vi "APcorrect.vi"(5 "EN_AP":dbl, 7 "c":dbl[](array[numeric]), 8 "error in":errorcluster, 10 "inputData":cdb[](array[numeric]), 11 "Path In":path) -> (0 "error out":errorcluster, 2 "out_data":cdb[](array[numeric]), 3 "Path Out":path)   [LabVIEW 2015]
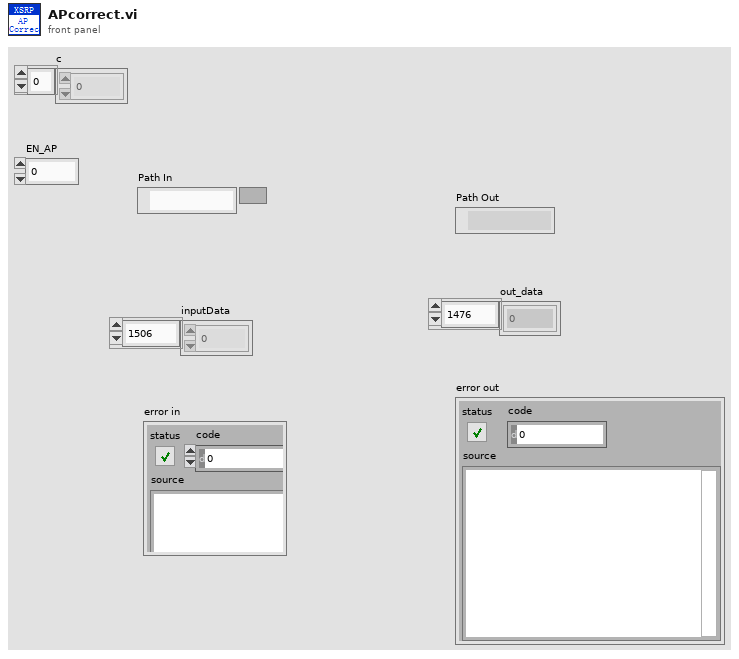
[diagram p1: front panel]
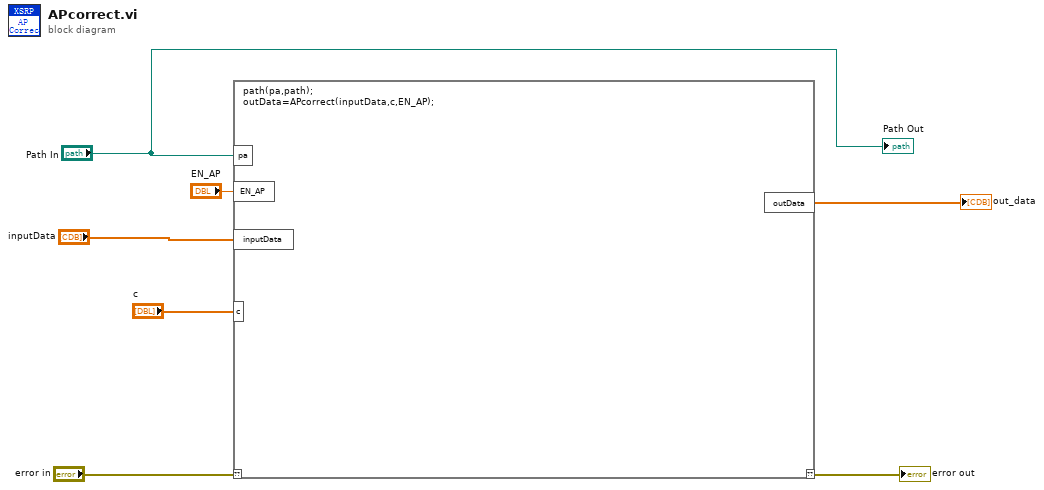
[diagram p0: block diagram]
diagram:
  n1 = script code="path(pa,path);\noutData=APcorrect(inputData,c,EN_AP);"("??"="error in", "pa"="Path In", "inputData"="inputData", "c"="c", "EN_AP"="EN_AP") -> ("??"=→"error out":errorcluster, "outData"=→"out_data":cdb[])
  "Path Out" <- "Path In"
